vi "RX_logic.vi"(0 "Settings":T3, 5 "Rx":bool) -> (4 "Busy":bool, 6 "RX_reply":T2, 10 "Rx_data":u16 format="%.0x", 15 "RX_State":T1)   [LabVIEW 2015, in "UART_Firmware.lvlib"]
uses:
  UART_Firmware.lvlib
  Settings.ctl
  Parity.ctl
  StopBits.ctl
  UART_Response.ctl
  RX_State.ctl
  RX_State_data.ctl
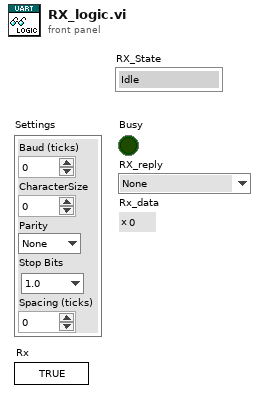
[diagram p1: front panel]
types:
  T1 = typedef "UART_Firmware.lvlib/RX_State.ctl" = enum16{"Idle", "FindCenterStart", "Character", "Parity", "Stop"}
  T2 = typedef "UART_Firmware.lvlib/UART_Response.ctl" = enum8{"None", "Rx", "BaudHighAck", "BaudLowAck", "CharSizeAck", "ParityAck", "StopBitsAck", "SpacingHighAck", "SpacingLowAck", "ParityError", "FrameError"}
  T3 = typedef "UART_Firmware.lvlib/Settings.ctl" = cluster{"Baud (ticks)":u32, "CharacterSize":u8, "Parity":T4, "Stop Bits":T5, "Spacing (ticks)":u32}
  T4 = typedef "UART_Firmware.lvlib/Parity.ctl" = enum8{"None", "Even", "Odd"}
  T5 = typedef "UART_Firmware.lvlib/StopBits.ctl" = enum8{"1.0", "1.5", "2.0"}
  T6 = typedef "UART_Firmware.lvlib/RX_State_data.ctl" = cluster{"Character":u16, "CharCount":u8, "Parity":bool, "RX_Reply":T2}
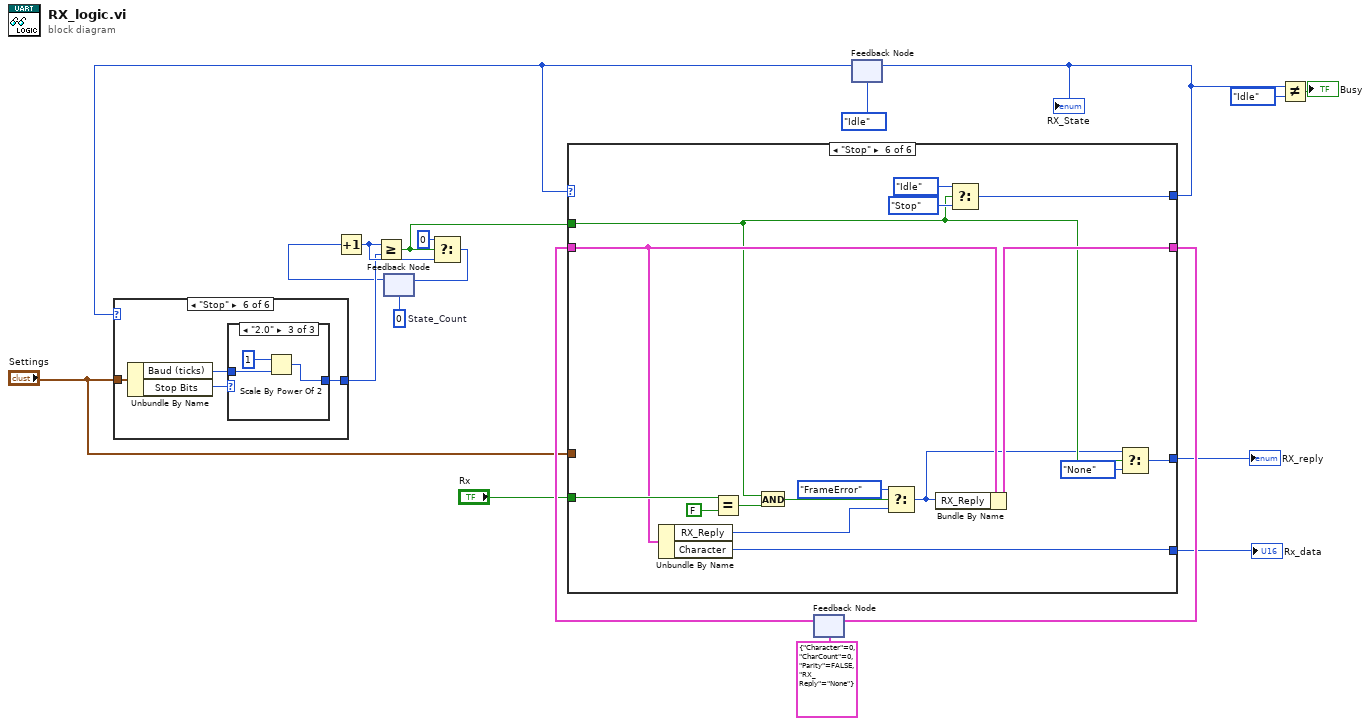
[diagram p0: block diagram]
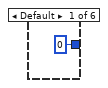
[diagram p2: hidden frame]
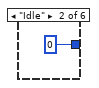
[diagram p3: hidden frame]
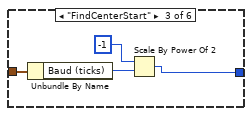
[diagram p4: hidden frame]
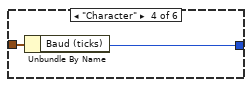
[diagram p5: hidden frame]
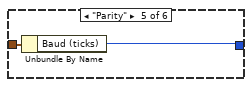
[diagram p6: hidden frame]
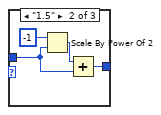
[diagram p8: hidden frame]
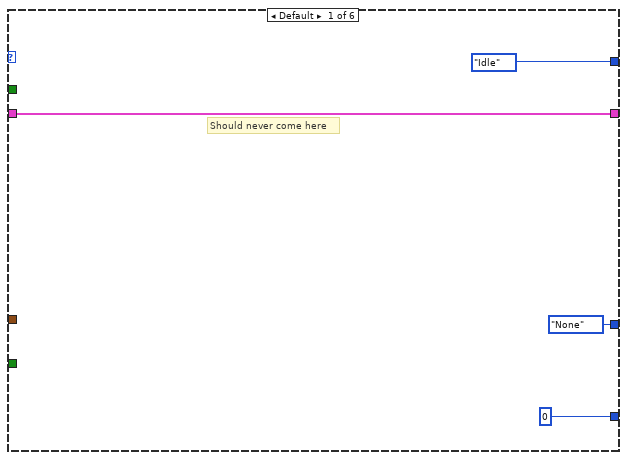
[diagram p9: hidden frame]
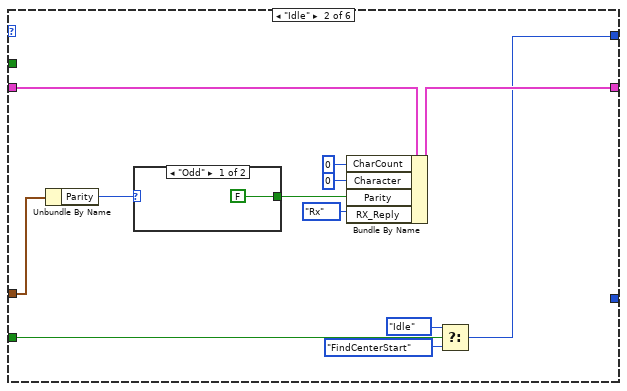
[diagram p10: hidden frame]
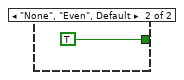
[diagram p11: hidden frame]
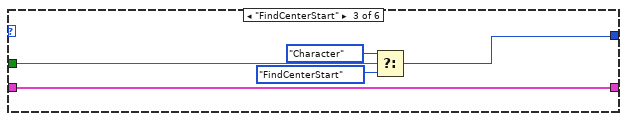
[diagram p12: hidden frame]
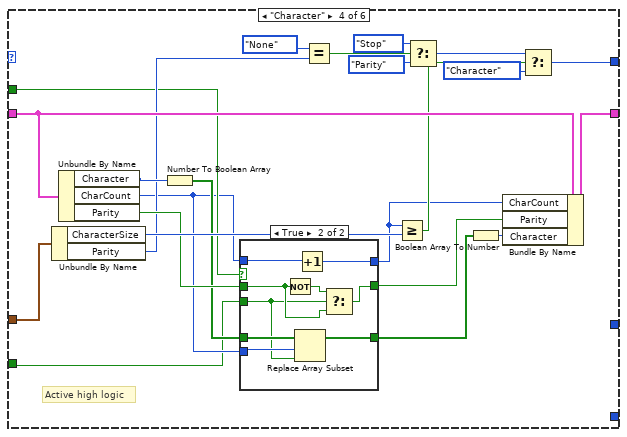
[diagram p13: hidden frame]
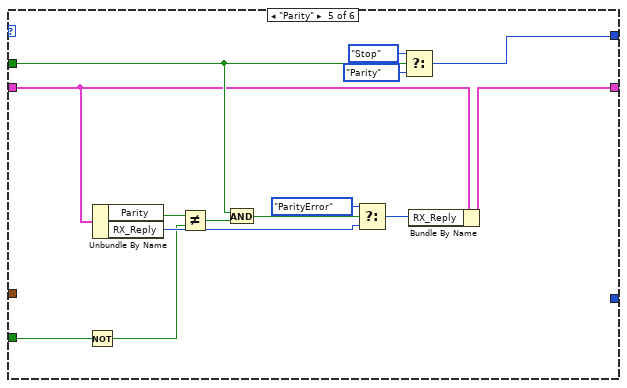
[diagram p15: hidden frame]
diagram:
  w13 = u32 0  # State_Count
  n1 = feedback #1(w13) -> (w12:u32)
  n2 = Increment(x=w12) -> (x+1=w16:u32)
  n3 = feedback #2(T6 {"Character"=0, "CharCount"=0, "Parity"=FALSE, "RX_Reply"=enum."None"} ("RX_State_Data")) -> (w10:T6)
  n4 = feedback #3(RX_State."Idle" ("RX_State")) -> (w3:T1)
  n5 = case shown="\"Stop\"" w3 {
    tunnel: "Settings" -> [_ _ w25 w27 w29 w33]
    tunnel: [u32 0 ("y") u32 0 ("y") w22 w26 w28 w30] -> w14
    frame Default {
    }
    frame "Idle" {
    }
    frame "FindCenterStart" {
      n6 = Unbundle By Name(w25) -> ("Baud (ticks)"=w24:u32)
      n7 = Scale By Power Of 2(n=-1, x=w24) -> (x*2^n=w22:u32)
    }
    frame "Character" {
      n8 = Unbundle By Name(w27) -> ("Baud (ticks)"=w26:u32)
    }
    frame "Parity" {
      n9 = Unbundle By Name(w29) -> ("Baud (ticks)"=w28:u32)
    }
    frame "Stop" {
      n10 = Unbundle By Name(w33) -> ("Baud (ticks)"=w31:u32, "Stop Bits"=w32:T5)
      n11 = case shown="\"2.0\"" w32 {
        tunnel: w31 -> [w34 w35 w41]
        tunnel: [w34 w37 w39] -> w30
        frame "1.0", Default {
        }
        frame "1.5" {
          n12 = Scale By Power Of 2(n=-1, x=w35) -> (x*2^n=w36:u32)
          n13 = Add(x=w36, y=w35) -> (x+y=w37:u32)
        }
        frame "2.0" {
          n14 = Scale By Power Of 2(n=1, x=w41) -> (x*2^n=w39:u32)
        }
      }
    }
  }
  n15 = Greater Or Equal?(x=w16, y=w14) -> (x >= y?=w15:bool)
  n16 = Select(t=u32 0 ("State_Count"), s=w15, f=w16) -> (s? t:f=w11:u32)
  n17 = feedback-in #1(w11) -> ()
  n18 = case shown="\"Stop\"" w3 {
    tunnel: w10 -> [w45 w57 w63 w85 w103 w120]
    tunnel: [RX_State."Idle" ("RX_State") w47 w64 w87 w113 w129] -> w18
    tunnel: "Settings" -> [_ w54 _ w84 _ _]
    tunnel: [w45 w56 w63 w86 w102 w119] -> w19
    tunnel: w15 -> [_ _ w62 w74 w108 w117]
    tunnel: "Rx" -> [_ w50 _ w65 w101 w126]
    tunnel: [u16 0 _ _ _ _ w118] -> w4
    tunnel: [UART_Response."None" ("f") _ _ _ _ w114] -> w2
    frame Default {
      # "Should never come here"
    }
    frame "Idle" {
      n19 = Unbundle By Name(w54) -> ("Parity"=w53:T4)
      n20 = case shown="\"Odd\"" w53 {
        tunnel: [FALSE TRUE] -> w52
        frame "Odd" {
        }
        frame "None", "Even", Default {
        }
      }
      n21 = Bundle By Name(cluster=w57, "CharCount"=u8 0 ("PayloadCount"), "Character"=u16 0, "Parity"=w52, "RX_Reply"=UART_Response."Rx") -> (w56:T6)
      n22 = Select(t=RX_State."Idle" ("RX_State"), s=w50, f=RX_State."FindCenterStart" ("RX_State")) -> (s? t:f=w47:T1)
    }
    frame "FindCenterStart" {
      n23 = Select(t=RX_State."Character" ("RX_State"), s=w62, f=RX_State."FindCenterStart") -> (s? t:f=w64:T1)
    }
    frame "Character" {
      # "Active high logic"
      n24 = Unbundle By Name(w84) -> ("CharacterSize"=w82:u8, "Parity"=w78:T4)
      n25 = Unbundle By Name(w85) -> ("Character"=w83:u16, "CharCount"=w67:u8, "Parity"=w80:bool)
      n26 = Number To Boolean Array(number=w83) -> (Boolean array=w70:bool[])
      n27 = case shown="True" w74 {
        tunnel: w80 -> [w90 w98]
        tunnel: [w90 w97] -> w79
        tunnel: w65 -> [_ w91]
        tunnel: w70 -> [w89 w96]
        tunnel: w67 -> [_ w95]
        tunnel: [w89 w94] -> w69
        tunnel: w67 -> [w88 w93]
        tunnel: [w88 w92] -> w66
        frame False {
        }
        frame True {
          n28 = Not(x=w98) -> (.not. x?=w99:bool)
          n29 = Replace Array Subset(array=w96, new element=w91, index=w95) -> (w94:bool[])
          n30 = Increment(x=w93) -> (x+1=w92:u8)
          n31 = Select(t=w99, s=w91, f=w98) -> (s? t:f=w97:bool)
        }
      }
      n32 = Equal?(x=Parity."None", y=w78) -> (x = y?=w76:bool)
      n33 = Greater Or Equal?(x=w66, y=w82) -> (x >= y?=w81:bool)
      n34 = Select(t=RX_State."Stop" ("RX_State"), s=w76, f=RX_State."Parity" ("RX_State")) -> (s? t:f=w75:T1)
      n35 = Boolean Array To Number(Boolean array=w69) -> (number=w68:u16)
      n36 = Bundle By Name(cluster=w85, "CharCount"=w66, "Parity"=w79, "Character"=w68) -> (w86:T6)
      n37 = Select(t=w75, s=w81, f=RX_State."Character" ("RX_State")) -> (s? t:f=w87:T1)
    }
    frame "Parity" {
      n38 = Not(x=w101) -> (.not. x?=w100:bool)
      n39 = Unbundle By Name(w103) -> ("Parity"=w110:bool, "RX_Reply"=w106:T2)
      n40 = Not Equal?(x=w110, y=w100) -> (x != y?=w109:bool)
      n41 = And(x=w108, y=w109) -> (x .and. y?=w107:bool)
      n42 = Select(t=UART_Response."ParityError", s=w107, f=w106) -> (s? t:f=w104:T2)
      n43 = Select(t=RX_State."Stop" ("RX_State"), s=w108, f=RX_State."Parity" ("RX_State")) -> (s? t:f=w113:T1)
      n44 = Bundle By Name(cluster=w103, "RX_Reply"=w104) -> (w102:T6)
    }
    frame "Stop" {
      n45 = Unbundle By Name(w120) -> ("RX_Reply"=w121:T2, "Character"=w118:u16)
      n46 = Equal?(x=w126, y=FALSE) -> (x = y?=w124:bool)
      n47 = And(x=w117, y=w124) -> (x .and. y?=w122:bool)
      n48 = Select(t=UART_Response."FrameError", s=w122, f=w121) -> (s? t:f=w116:T2)
      n49 = Bundle By Name(cluster=w120, "RX_Reply"=w116) -> (w119:T6)
      n50 = Select(t=RX_State."Idle" ("RX_State"), s=w117, f=RX_State."Stop" ("RX_State")) -> (s? t:f=w129:T1)
      n51 = Select(t=w116, s=w117, f=UART_Response."None") -> (s? t:f=w114:T2)
    }
  }
  "Rx_data" <- w4
  "RX_reply" <- w2
  "RX_State" <- w18
  n52 = feedback-in #2(w19) -> ()
  n53 = feedback-in #3(w18) -> ()
  n54 = Not Equal?(x=w18, y=RX_State."Idle" ("RX_State")) -> (x != y?=→"Busy":bool)
